vi "PyLoN_SRS.vi"() -> ()   [LabVIEW 2014]
uses:
  C:/Users/wrsilva/Desktop/Labview VIs/PIXIS_TEST/SITK_Labview/Examples70_2_2_0_1/RS Pixis/MaxY.vi
  C:/Users/wrsilva/Desktop/Labview VIs/PIXIS_TEST/SITK_Labview/Examples70_2_2_0_1/RS Pixis/MaxX.vi
panel:
  in  "?":bool
  in  "?":T1(tab)
  in  "Shutter State":u16(ring)=2 items=["Always Close", "Open Each Exposure", "Open Until Finish", "Open waiting for triger"]
  in  "Trigger Edge":u16(ring) items=["Positive", "Negative"]
  in  "Timing Mode":u16(ring) items=["Free Run", "Triger First", "EXt Sync", "Bulb Mode", "Variable Mode", "Flash Mode"]
  in  "ADC Speed":u16(ring)=2 items=["ADC Slow", "ADC Fast", "Default"]
  in  "ADC Gain":u16(ring) items=["ADC Low", "ADC High"]
  in  "Temperature":dbl=-100.0 caption="SET Temperature" format="%.2f"
  in  "skip serial  reg clean":dbl=1.0 format="%.2f"
  in  "Vertical timing 2":dbl=3.2
  out "Vertical timing":dbl
  in  "Read Out port":i32=4 min=-1 step=1
  in  "?":T2={"X start"=0, "X end"=1023, "X Binning/Grouping"=1, "Y start"=0, "Y end"=1, "Y Binning/Grouping"=1}
  in  "Exposure Time (s)":dbl=0.004 min=0.0 step=0.001 format="%.3f"
  in  "?":bool
  in  "?":bool
  out "?":u16[](graph)
  in  "PyLonN Error In":errorcluster
  out "PyLoN Error Out":errorcluster
  out "PyLoN Ready":bool
  out "PyLoN \nTemperature":dbl
  # "REGION OF INTEREST"
  # "TRIGGER"
  # "ADC"
  # "SHUTTER"
  # "CUSTOM CHIP"
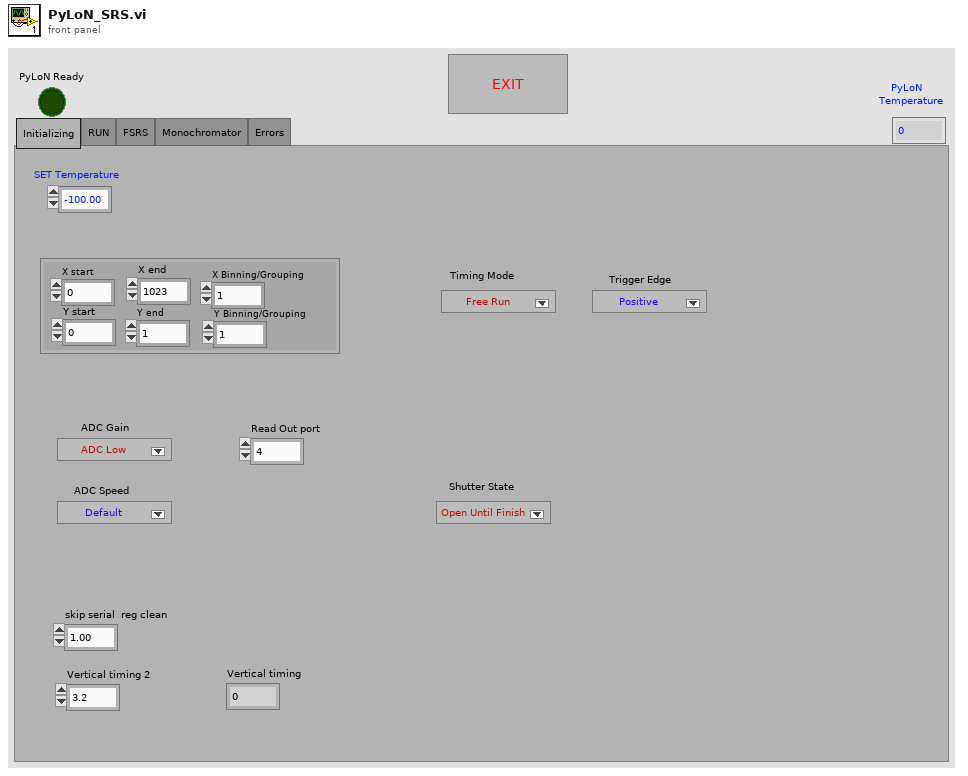
[diagram p1: front panel]
types:
  T1 = enum32{"Initializing", "RUN", "FSRS", "Monochromator", "Errors"}
  T2 = cluster{"X start":u32, "X end":u32, "X Binning/Grouping":u32, "Y start":u32, "Y end":u32, "Y Binning/Grouping":u32}
  T3 = cluster{"acquire focus mode":u32, "Exposure Time (s)":dbl, i32, "Software accumulation":u32}
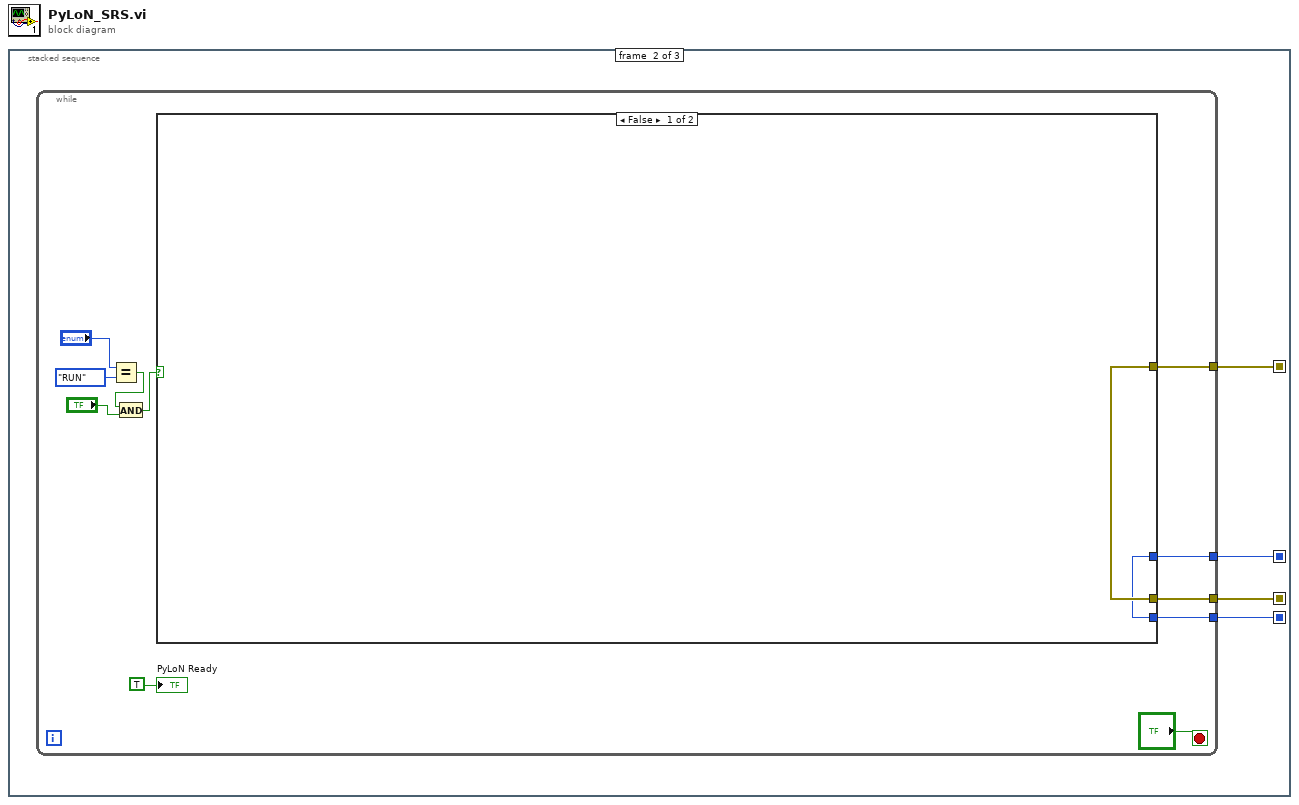
[diagram p0: block diagram]
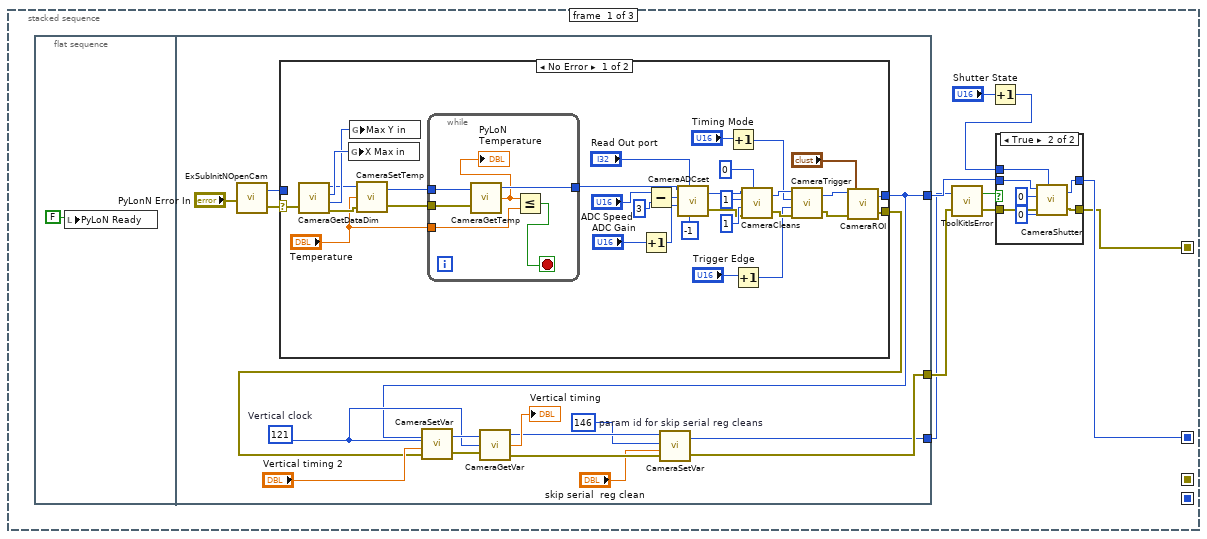
[diagram p2: hidden frame]
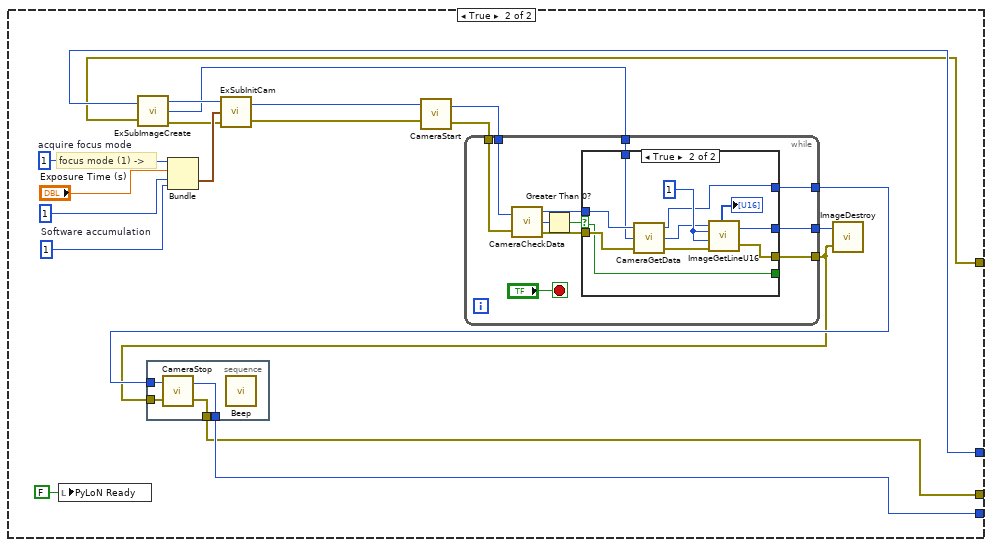
[diagram p5: hidden frame]
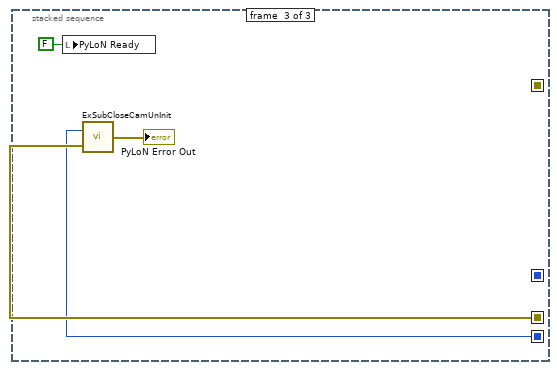
[diagram p7: hidden frame]
diagram:
  n1 = stacked-sequence {
    seq-local: [w4 _ _] -> [_ w78 _]
    seq-local: [w7 _ _] -> [_ w79 _]
    seq-local: [_ w77 _] -> [_ _ w145]
    seq-local: [_ w76 _] -> [_ _ w144]
    frame #0 {
      n2 = flat-sequence {
        tunnel: [w18] -> w9
        tunnel: [w14] -> w6
        tunnel: [w11] -> w3
        frame #0 {
          n3 = local write "PyLoN Ready"(FALSE ("PyLoN Ready")) -> ()
        }
        frame #1 {
          w12 = 146  # param id for skip serial reg cleans
          w21 = u32 121  # Vertical clock
          n4 = call "ExSubInitNOpenCam.vi"("error in (no error)"="PyLonN Error In") -> ("Camera Handle"=w24:u32, "error out"=w25:errorcluster)
          n5 = case shown="No Error" w25 {
            selector: w25 -> [w42 w66]
            tunnel: w24 -> [_ w65]
            tunnel: [w37 w65] -> w18
            tunnel: [w36 w66] -> w17
            frame No Error {
              n6 = call <userlib>:"CameraGetDataDim.vi"("error in"=w42) -> ("Camera Handle"=w56:u32, "Xdim"=w58:u32, "Ydim"=w57:u32, "error out"=w55:errorcluster)  [unwired: 1 in]
              n7 = global write "MaxX.vi" "X Max in"(w58) -> ()
              n8 = global write "MaxY.vi" "Max Y in"(w57) -> ()
              n9 = call <userlib>:"CameraSetTemp.vi"("error in (no error)"=w55, "Temperature"="Temperature", "Camera Handle"=w56) -> ("error out"=w40:errorcluster, "Camera Handle"=w41:u32)
              n10 = while {
                tunnel: w41 -> [w64]
                tunnel: w40 -> [w63]
                tunnel: "Temperature" -> [w62]
                tunnel: [w60] -> w38
                stop <- w61 stop-if-true
                n11 = call <userlib>:"CameraGetTemp.vi"("Camera Handle"=w64, "error in (no error)"=w63) -> ("Camera Handle"=w60:u32, "Temperature"=w59:dbl)  [unwired: 1 out]
                "PyLoN \nTemperature" <- w59
                n12 = Less Or Equal?(x=w59, y=w62) -> (x <= y?=w61:bool)
              }
              n13 = Increment(x="ADC Gain") -> (x+1=w53:u16)
              n14 = Subtract(x="ADC Speed", y=u16 3) -> (x-y=w34:u16)
              n15 = call <userlib>:"CameraADCset.vi"("ADC offset"=-1, "Read Out port"="Read Out port", "ADC Gain"=w53, "ADC Speed"=w34, "Camera Handle"=w38) -> ("error out"=w45:errorcluster, "Camera Handle"=w51:u32)  [unwired: 1 in]
              n16 = Increment(x="Timing Mode") -> (x+1=w29:u16)
              n17 = Increment(x="Trigger Edge") -> (x+1=w27:u16)
              n18 = call <userlib>:"CameraCleans.vi"("Camera Handle"=w51, "Number of Clears"=u32 1, "Number of Strips Per Clear"=u32 1, "error in"=w45, "Continuous Clears"=u32 0) -> ("Camera Handle"=w50:u32, "error out"=w44:errorcluster)
              n19 = call <userlib>:"CameraTrigger.vi"("error in"=w44, "Trigger Edge"=w27, "Timing Mode"=w29, "Camera Handle"=w50) -> ("error out"=w43:errorcluster, "Camera Handle"=w49:u32)
              n20 = call <userlib>:"CameraROI.vi"("error in"=w43, "ROI Params"="?", "Camera Handle"=w49) -> ("error out"=w36:errorcluster, "Camera Handle"=w37:u32)  [unwired: 1 in]
            }
            frame Error {
            }
          }
          n21 = call <userlib>:"CameraSetVar.vi"("error in"=w17, "Value"="Vertical timing 2", "Parameter ID"=w21, "Camera Handle"=w18) -> ("error out"=w20:errorcluster, "CameraHandle"=w22:u32)
          n22 = call <userlib>:"CameraGetVar.vi"("error in"=w20, "Parameter ID"=w21, "Camera Handle"=w22) -> ("error out"=w15:errorcluster, "Value"=→"Vertical timing":dbl, "Camera Handle"=w16:u32)
          n23 = call <userlib>:"CameraSetVar.vi"("error in"=w15, "Value"="skip serial  reg clean", "Parameter ID"=w12, "Camera Handle"=w16) -> ("error out"=w14:errorcluster, "CameraHandle"=w11:u32)
        }
      }
      n24 = call <userlib>:"ToolKitIsError.vi"("error in"=w6, "Reserved"=w3) -> ("error out"=w5:errorcluster, "Error Flag"=w8:bool)
      n25 = Increment(x="Shutter State") -> (x+1=w1:u16)
      n26 = case shown="True" w8 {
        tunnel: w9 -> [w68 w73]
        tunnel: [w67 w72] -> w4
        tunnel: [w68 w71] -> w7
        tunnel: w5 -> [w67 w70]
        tunnel: w1 -> [_ w69]
        frame False {
        }
        frame True {
          n27 = call <userlib>:"CameraShutter.vi"("Camera Handle"=w73, "Shutter Comp Time: Pre Open"=u32 0, "Shutter Comp Time: Post Open"=u32 0, "error in"=w70, "Shutter State"=w69) -> ("Camera Handle"=w71:u32, "error out"=w72:errorcluster)
        }
      }
    }
    frame #1 {
      n28 = while {
        tunnel: w79 -> [w90]
        tunnel: w78 -> [w89]
        tunnel: [w88] -> w77
        tunnel: [w87] -> w76
        stop <- "?" stop-if-true
        n29 = Equal?(x="?", y=T1."RUN") -> (x = y?=w84:bool)
        n30 = And(x=w84, y="?") -> (x .and. y?=w82:bool)
        n31 = case shown="False" w82 {
          tunnel: w90 -> [w91 w112]
          tunnel: w89 -> [w92 w111]
          tunnel: [w91 w110] -> w87
          tunnel: [w92 w109] -> w88
          frame False {
          }
          frame True {
            w107 = u32 1  # acquire focus mode
            w106 = u32 1  # Software accumulation
            # "focus mode (1) ->"
            n32 = local write "PyLoN Ready"(FALSE ("PyLoN Ready")) -> ()
            n33 = call "ExSubImageCreate.vi"("Camera Handle"=w112, "error in (no error)"=w111) -> ("Camera Handle"=w105:u32, "Data Handle"=w99:u32, "error out"=w104:errorcluster)
            n34 = Bundle("acquire focus mode"=w107, "Exposure Time (s)"="Exposure Time (s)", 1, "Software accumulation"=w106) -> (w108:T3)  [unwired: 1 in]
            n35 = call "ExSubInitCam.vi"("error in (no error)"=w104, "Camera Information"=w108, "Camera Handle"=w105) -> ("error out"=w103:errorcluster, "Camera Handle"=w102:u32)
            n36 = call <userlib>:"CameraStart.vi"("error in"=w103, "Camera Handle"=w102) -> ("error out"=w101:errorcluster, "Camera Handle"=w100:u32)
            n37 = while {
              tunnel: [w122] -> w98
              tunnel: [w121] -> w96
              tunnel: [w120] -> w97
              tunnel: w101 -> [w119]
              tunnel: w100 -> [w118]
              tunnel: w99 -> [w117]
              stop <- "?" stop-if-true
              n38 = call <userlib>:"CameraCheckData.vi"("Camera Handle"=w118, "error in"=w119) -> ("Camera Handle"=w125:u32, "Number Of Frames Available"=w127:i32, "error out"=w124:errorcluster)
              n39 = Greater Than 0?(x=w127) -> (x > 0?=w126:bool)
              n40 = case shown="True" w126 {
                selector: w126 -> [w130 w140]
                tunnel: w125 -> [w128 w142]
                tunnel: w124 -> [w131 w141]
                tunnel: [w130 w140] -> _
                tunnel: [w131 w138] -> w121
                tunnel: w117 -> [w129 w132]
                tunnel: [w129 w136] -> w122
                tunnel: [w128 w135] -> w120
                frame False {
                }
                frame True {
                  w137 = 1
                  n41 = call <userlib>:"CameraGetData.vi"("error in"=w141, "Data Handle"=w132, "Camera Handle"=w142) -> ("error out"=w134:errorcluster, "Data Handle"=w133:u32, "Camera Handle"=w135:u32)
                  n42 = call <userlib>:"ImageGetLineU16.vi"("Data Handle"=w133, "Y Position"=w137, "Z Position"=w137, "error in"=w134) -> ("Array u16"=→"?":u16[], "Data Handle"=w136:u32, "error out"=w138:errorcluster)
                }
              }
            }
            n43 = stacked-sequence {
              tunnel: w96 -> [w116]
              tunnel: w97 -> [w115]
              tunnel: [w114] -> w109
              tunnel: [w113] -> w110
              frame #0 {
                n44 = call <userlib>:"CameraStop.vi"("error in"=w116, "Camera Handle"=w115) -> ("error out"=w114:errorcluster, "Camera Handle"=w113:u32)
                n45 = call <vilib>:"Beep.vi"() -> ()  [unwired: 12 in]
              }
            }
            n46 = call <userlib>:"ImageDestroy.vi"("error in"=w96, "Data handle"=w98) -> ()  [unwired: 1 out]
          }
        }
        "PyLoN Ready" <- TRUE
      }
    }
    frame #2 {
      n47 = local write "PyLoN Ready"(FALSE ("PyLoN Ready")) -> ()
      n48 = call "ExSubCloseCamUnInit.vi"("error in (no error)"=w145, "Camera Handle"=w144) -> ("error out"=→"PyLoN Error Out":errorcluster)
    }
  }
